vi "SetStreamMode.vi"(7 "Timeout (ms)":u32=2000, 8 "Error In":errorcluster, 10 "Mode":T1, 11 "Sierra M100 In":refnum<visa-resource-name>) -> (0 "Error Out":errorcluster, 2 "Set?":bool, 3 "Sierra M100 Out":refnum<visa-resource-name>)   [LabVIEW 2012, in "Sierra-M100.lvlib"]
doc: "This VI sets the streaming mode. The streamming on is either \"on\", \"off\", or \"echo\". In \"on\" data will continually be loaded onto the serial communication. For this reason, the \"Initialize\" VI disables the streaming mode."
uses:
  Sierra-M100.lvlib
  Controls/StreamMode.ctl
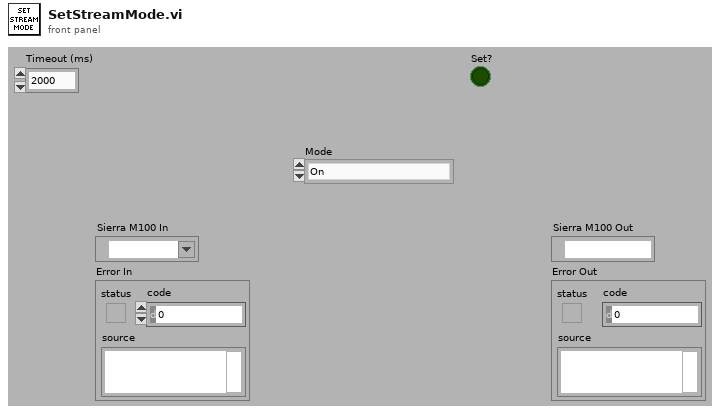
[diagram p1: front panel]
types:
  T1 = typedef "Sierra-M100.lvlib/StreamMode.ctl" = enum16{"On", "Off", "Echo"}
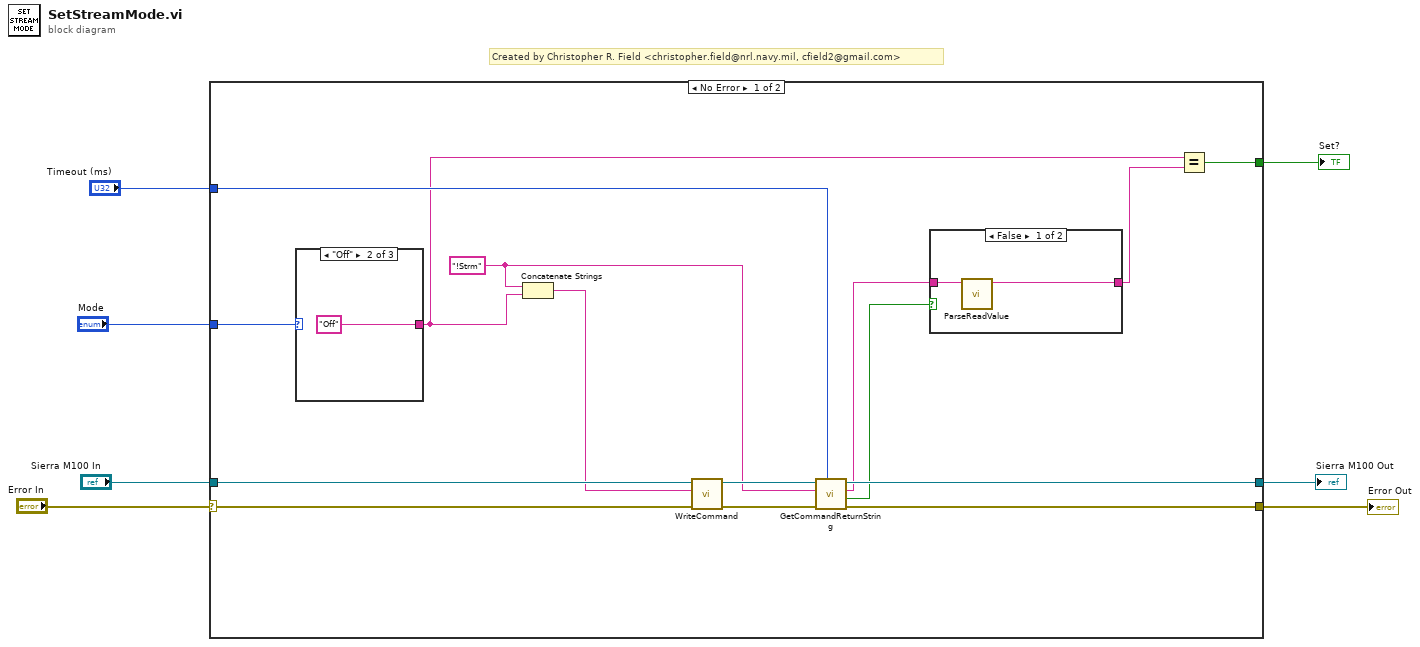
[diagram p0: block diagram]
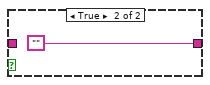
[diagram p2: hidden frame]
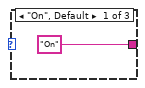
[diagram p3: hidden frame]
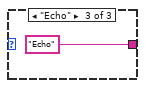
[diagram p4: hidden frame]
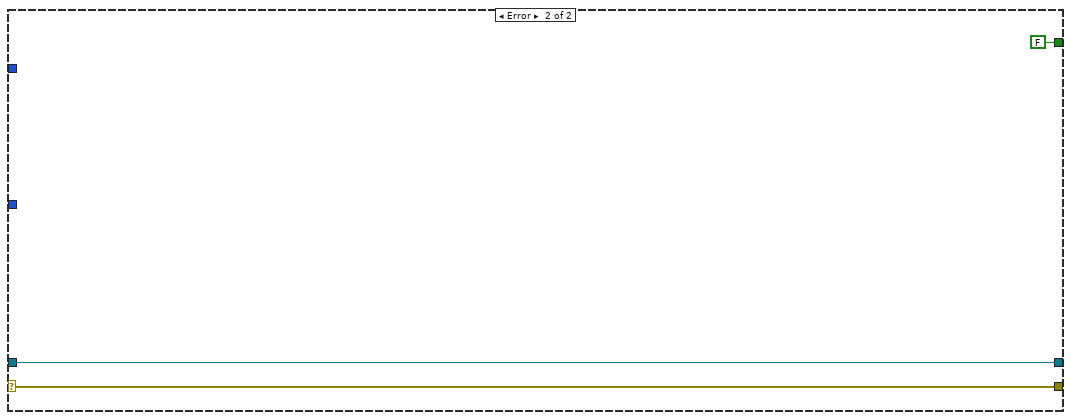
[diagram p5: hidden frame]
diagram:
  # "Created by Christopher R. Field <christopher.field@nrl.navy.mil, cfield2@gmail.com>"
  n1 = case shown="No Error" "Error In" {
    selector: "Error In" -> [w8 w30]
    tunnel: "Mode" -> [w22 _]
    tunnel: "Sierra M100 In" -> [w21 w31]
    tunnel: "Timeout (ms)" -> [w16 _]
    tunnel: [w15 w31] -> w4
    tunnel: [w14 w30] -> w3
    tunnel: [w9 FALSE] -> w2
    frame No Error {
      w18 = "!Strm"
      n2 = case shown="\"Off\"" w22 {
        tunnel: ["On" "Off" "Echo"] -> w10
        frame "On", Default {
        }
        frame "Off" {
        }
        frame "Echo" {
        }
      }
      n3 = Concatenate Strings(w18, w10) -> (w20:string)
      n4 = call "WriteCommand.vi"("Error In"=w8, "Command"=w20, "Smart Trak 2 In"=w21) -> ("Error Out"=w17:errorcluster, "Smart Trak 2 Out"=w19:refnum<visa-resource-name>)  [unwired: 5 in, 2 out]
      n5 = call "GetCommandReturnString.vi"("Timeout (ms)"=w16, "Error In"=w17, "Command"=w18, "Smart Trak 2 In"=w19) -> ("Error Out"=w14:errorcluster, "Timeout?"=w12:bool, "Return String"=w13:string, "Smart Trak 2 Out"=w15:refnum<visa-resource-name>)  [unwired: 4 in]
      n6 = case shown="False" w12 {
        tunnel: w13 -> [w24 _]
        tunnel: [w23 ""] -> w11
        frame False {
          n7 = call "ParseReadValue.vi"("Read Buffer"=w24) -> ("Value"=w23:string)  [unwired: 10 in]
        }
        frame True {
        }
      }
      n8 = Equal?(x=w10, y=w11) -> (x = y?=w9:bool)
    }
    frame Error {
    }
  }
  "Sierra M100 Out" <- w4
  "Error Out" <- w3
  "Set?" <- w2
